vi "Count photons with FPGA.vi"(8 "error in (no error)":errorcluster, 10 "Entrainment":bool) -> (0 "error out":errorcluster)   [LabVIEW 2013]
uses:
  <vilib>/DAQmx/write.llb/DAQmx Write (Digital Bool 1Line 1Point).vi
  <vilib>/DAQmx/read.llb/DAQmx Read (Digital Bool 1Line 1Point).vi
  <vilib>/DAQmx/miscellaneous.llb/DAQmx Fill In Error Info.vi
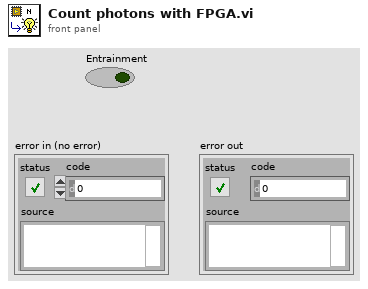
[diagram p1: front panel]
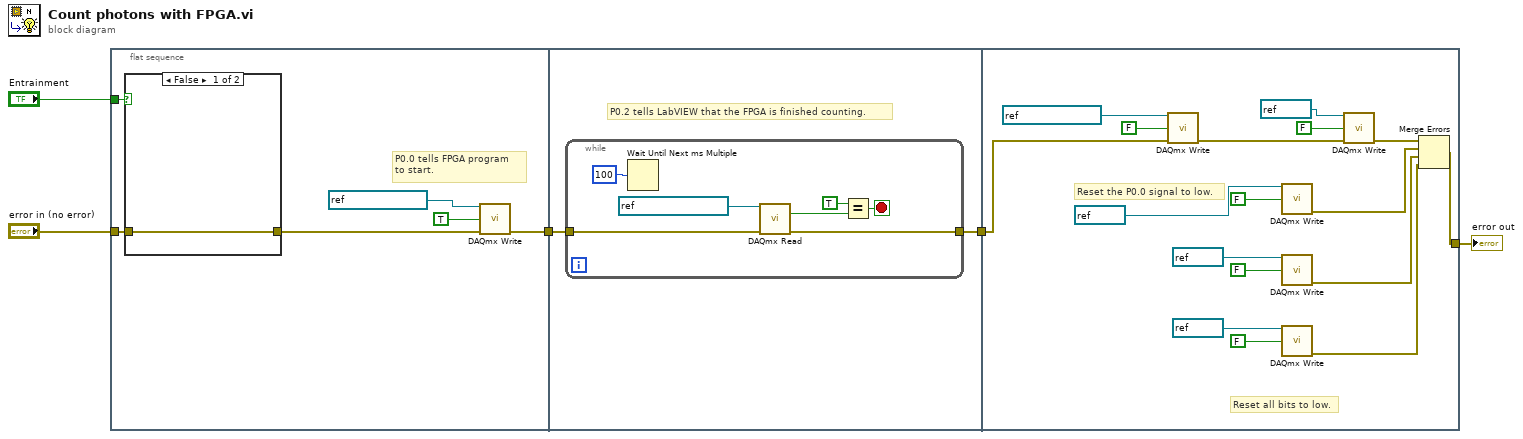
[diagram p0: block diagram]
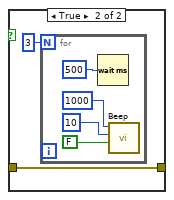
[diagram p2: hidden frame]
diagram:
  n1 = flat-sequence {
    tunnel: [w9] -> w5
    tunnel: "Entrainment" -> [w8]
    tunnel: "error in (no error)" -> [w6]
    tunnel: w5 -> [w20]
    tunnel: [w19] -> w4
    tunnel: [w28] -> w3
    tunnel: w4 -> [w34]
    frame #0 {
      # "P0.0 tells FPGA program \nto start."
      n2 = case shown="False" w8 {
        tunnel: w6 -> [w12 w13]
        tunnel: [w12 w13] -> w7
        frame False {
        }
        frame True {
          n3 = for {
            N: 3 -> [_]
            n4 = Wait (ms)(milliseconds to wait=u32 500) -> ()  [unwired: 1 out]
            n5 = call <vilib>:"Beep.vi"("use system alert? (T)"=FALSE, "duration (msec)"=u32 10, "frequency (Hz)"=u32 1000) -> ()  [unwired: 9 in]
          }
        }
      }
      n6 = call-poly <vilib>:"DAQmx Write.vi"("task/channels in"=refnum<k21> "LaserChannel", "data"=TRUE, "error in"=w7) -> ("error out"=w9:errorcluster)  [unwired: 10 in, 2 out]
    }
    frame #1 {
      # "P0.2 tells LabVIEW that the FPGA is finished counting."
      n7 = while {
        tunnel: w20 -> [w26]
        tunnel: [w25] -> w19
        stop <- w22 stop-if-true
        n8 = Wait Until Next ms Multiple(millisecond multiple=u32 100) -> ()  [unwired: 1 out]
        n9 = call-poly <vilib>:"DAQmx Read.vi"("task/channels in"=refnum<k21> "P02countSignal", "error in"=w26) -> ("data"=w23:bool, "error out"=w25:errorcluster)  [unwired: 11 in, 1 out]
        n10 = Equal?(x=TRUE, y=w23) -> (x = y?=w22:bool)
      }
    }
    frame #2 {
      # "Reset all bits to low."
      # "Reset the P0.0 signal to low."
      n11 = call-poly <vilib>:"DAQmx Write.vi"("task/channels in"=refnum<k21> "LaserChannel", "data"=FALSE, "error in"=w34) -> ("error out"=w33:errorcluster)  [unwired: 10 in, 2 out]
      n12 = call-poly <vilib>:"DAQmx Write.vi"("task/channels in"=refnum<k21> "BIT2", "data"=FALSE) -> ("error out"=w41:errorcluster)  [unwired: 11 in, 2 out]
      n13 = call-poly <vilib>:"DAQmx Write.vi"("task/channels in"=refnum<k21> "BIT3", "data"=FALSE) -> ("error out"=w40:errorcluster)  [unwired: 11 in, 2 out]
      n14 = call-poly <vilib>:"DAQmx Write.vi"("task/channels in"=refnum<k21> "BIT4", "data"=FALSE) -> ("error out"=w39:errorcluster)  [unwired: 11 in, 2 out]
      n15 = call-poly <vilib>:"DAQmx Write.vi"("task/channels in"=refnum<k21> "BIT1", "data"=FALSE, "error in"=w33) -> ("error out"=w42:errorcluster)  [unwired: 10 in, 2 out]
      n16 = Merge Errors(w42, w41, w40, w39) -> (w28:errorcluster)
    }
  }
  "error out" <- w3
